vi "Extract Latest.vi"(8 "Error":errorcluster, 10 "Raw Data Waveform":T1, 11 "((Pointer))":refnum<class "Absolute_Pointer.lvclass">) -> (0 "Error Out":errorcluster, 2 "Waveform Out":T1, 3 "((Pointer)) Out":refnum<class "Absolute_Pointer.lvclass">)   [LabVIEW 2024, in "Absolute_Pointer.lvclass"]
uses:
  Absolute_Pointer.lvclass
  Universal Controls/Waveform_Data.ctl
  _Pointer.lvclass
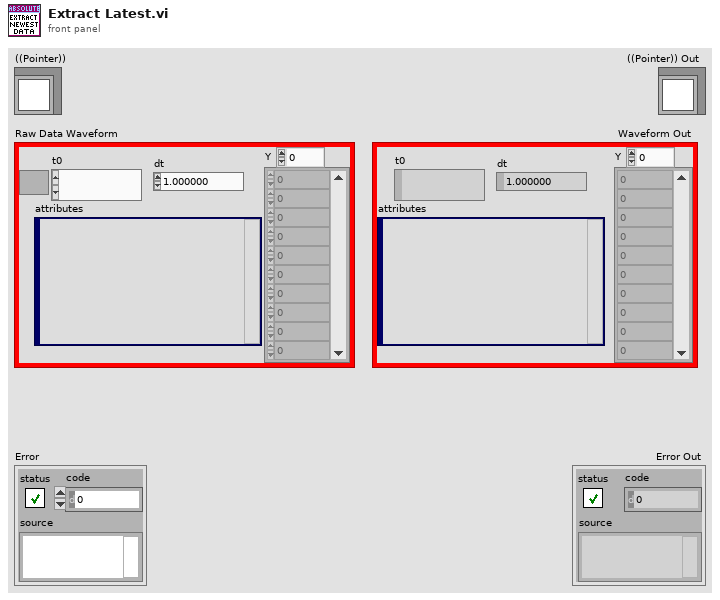
[diagram p1: front panel]
types:
  T1 = typedef "Waveform_Data.ctl" = waveform(dbl)
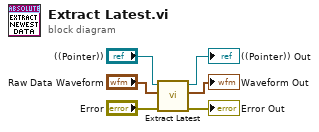
[diagram p0: block diagram]
diagram:
  n1 = call-parent "Extract Latest.vi"("Error"="Error", "Raw Data Waveform"="Raw Data Waveform", "((Pointer))"="((Pointer))") -> ("Error Out"=→"Error Out":errorcluster, "Waveform Out"=→"Waveform Out":T1, "((Pointer)) Out"=→"((Pointer)) Out":refnum<class "Absolute_Pointer.lvclass">)  [unwired: 6 in]
